vi "Obtain Hwnd.vi"(0 "LV RT in":refnum<class "LV RT.lvclass">, 5 "Parent Hwnd":i32, 11 "error in (no error)":errorcluster) -> (4 "LV RT out":refnum<class "LV RT.lvclass">, 15 "error out":errorcluster)   [LabVIEW 2016, in "LV RT.lvclass"]
uses:
  LV RT.lvclass
  D:/MDI Project/source code/Document/Child Classes/LV Doc/LV Doc.lvclass
  D:/MDI Project/source code/Document/Document.lvclass
  LV Doc.lvclass/LV Doc.ctl
  Document.lvclass/Document.ctl
  LV Doc.lvclass
  Document.lvclass
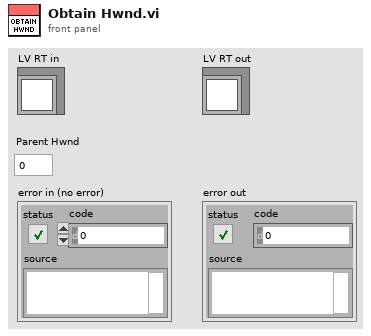
[diagram p1: front panel]
types:
  T1 = enum32{"Invalid", "Standard", "Closed", "Hidden", "Minimized", "Maximized"}
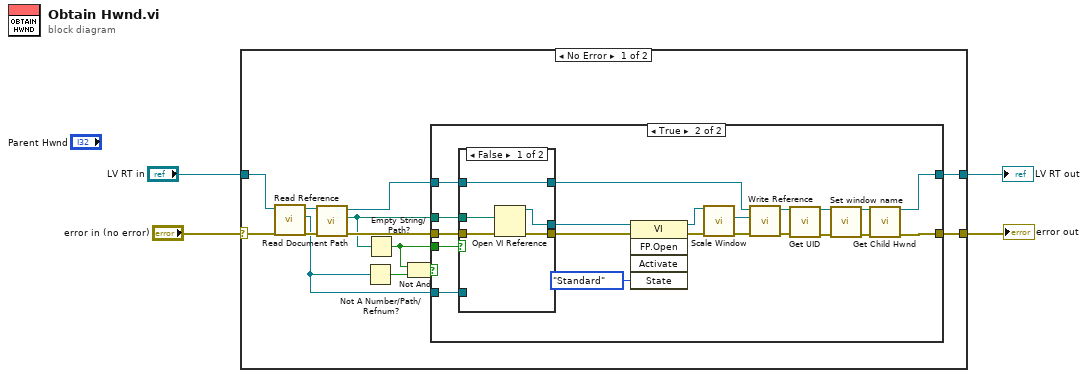
[diagram p0: block diagram]
diagram:
  n1 = case shown="No Error" "error in (no error)" {
    selector: "error in (no error)" -> [w12 w49]
    tunnel: [w17 w50] -> w4
    tunnel: [w16 w49] -> w3
    tunnel: "LV RT in" -> [w10 w50]
    frame No Error {
      n2 = call "Read Reference.vi"("error in (no error)"=w12, "LV Doc in"=w10) -> ("error out"=w11:errorcluster, "Reference"=w6:refnum<vi>, "LV Doc out"=w9:refnum<class "LV RT.lvclass">)  [unwired: 7 in]
      n3 = call "Read Document Path.vi"("error in (no error)"=w11, "Document in"=w9) -> ("error out"=w14:errorcluster, "Document Path"=w13:path, "Document out"=w15:refnum<class "LV RT.lvclass">)  [unwired: 7 in]
      n4 = Not A Number/Path/Refnum?(number/path/refnum=w6) -> (NaN/Path/Refnum?=w8:bool)
      n5 = Empty String/Path?(string/path=w13) -> (empty?=w5:bool)
      n6 = Not And(1:w8, 2:w5) -> (0:w7:bool)
      n7 = case shown="True" w7 {
        tunnel: [w18 w40] -> w17
        tunnel: [w19 w39] -> w16
        tunnel: w15 -> [w18 w21]
        tunnel: w14 -> [w19 w25]
        tunnel: w13 -> [_ w24]
        tunnel: w6 -> [_ w23]
        tunnel: w5 -> [_ w22]
        frame False {
        }
        frame True {
          n8 = case shown="False" w22 {
            tunnel: [w45 w47] -> w27
            tunnel: [w44 w48] -> w26
            tunnel: w25 -> [w43 w48]
            tunnel: w24 -> [w42 _]
            tunnel: w23 -> [_ w47]
            tunnel: w21 -> [w41 w46]
            tunnel: [w41 w46] -> w20
            frame False {
              n9 = Open VI Reference(vi path=w42, error in (no error)=w43) -> (vi reference=w45:refnum<vi>, error out=w44:errorcluster)  [unwired: 4 in]
            }
            frame True {
            }
          }
          n10 = invoke class="VI" method="FP.Open"(reference=w27, error in=w26, "State"=T1."Standard") -> (reference out=w30:refnum<vi>, error out=w29:errorcluster)  [unwired: 2 in, 3 out]
          n11 = call "Scale Window.vi"("VI in"=w30, "error in (no error)"=w29) -> ("VI out"=w32:refnum<vi>, "error out"=w31:errorcluster)  [unwired: 12 in]
          n12 = call "Write Reference.vi"("error in (no error)"=w31, "Reference"=w32, "LV Doc in"=w20) -> ("error out"=w35:errorcluster, "LV Doc out"=w36:refnum<class "LV RT.lvclass">)  [unwired: 7 in]
          n13 = call "Get UID.vi"("LV Doc.lvclass"=w36, "error in (no error)"=w35) -> ("LV Doc.lvclass"=w34:refnum<class "LV RT.lvclass">, "error out"=w37:errorcluster)  [unwired: 12 in]
          n14 = call "Set window name.vi"("LV Doc.lvclass"=w34, "error in (no error)"=w37) -> ("LV Doc.lvclass"=w33:refnum<class "LV RT.lvclass">, "error out"=w38:errorcluster)  [unwired: 12 in]
          n15 = call "Get Child Hwnd.vi"("LV Doc.lvclass"=w33, "Error in"=w38) -> ("LV Doc.lvclass"=w40:refnum<class "LV RT.lvclass">, "Error Out"=w39:errorcluster)  [unwired: 12 in]
        }
      }
    }
    frame Error {
    }
  }
  "LV RT out" <- w4
  "error out" <- w3
